vi "ACQUIS_BASE2_2015.vi"(1 "sample mode":i32(ring)=10178 items=["Finite Samples"=10178, "Continuous Samples"=10123, "Hardware Timed Single Point"=12522], 2 "Campioni al secondo":sgl=50000.0, 3 "Fondo Scala":enum16{"10", "5", "0.5", "0.05"}(ring), 4 "physical channels":tag="Dev1/ai0:1", 5 "input terminal configuration":i32(ring)=10083 items=["default"=-1, "RSE"=10083, "NRSE"=10078, "Differential"=10106, "Pseudodifferential"=12529], 6 "Durata (secondi)":dbl=0.05 format="%#.5f") -> ()   [LabVIEW 2014]
doc: "AnalogInput versione 7\nVersione base (2 canale) per schede 6024E\n(per le 6221 occorre cambiare il vettore Fondo scala)\nFM & ADL 2007\nsalva anche i dati (due colonne con solo Y1 e Y2 dopo una riga di intestazione\ngenn 2013"
uses:
  <vilib>/DAQmx/read.llb/DAQmx Read (Analog 2D DBL NChan NSamp).vi
  <vilib>/DAQmx/create/channels.llb/DAQmx Create Channel (AI-Voltage-Basic).vi
  <vilib>/DAQmx/configure/timing.llb/DAQmx Timing (Sample Clock).vi
  <vilib>/DAQmx/miscellaneous.llb/DAQmx Fill In Error Info.vi
panel:
  out "Grafico Dati":dbl[][](graph)
  in  "SALVA I DATI SU FILE":bool=TRUE caption="ON\nOFF"
  # "NO\nSI"
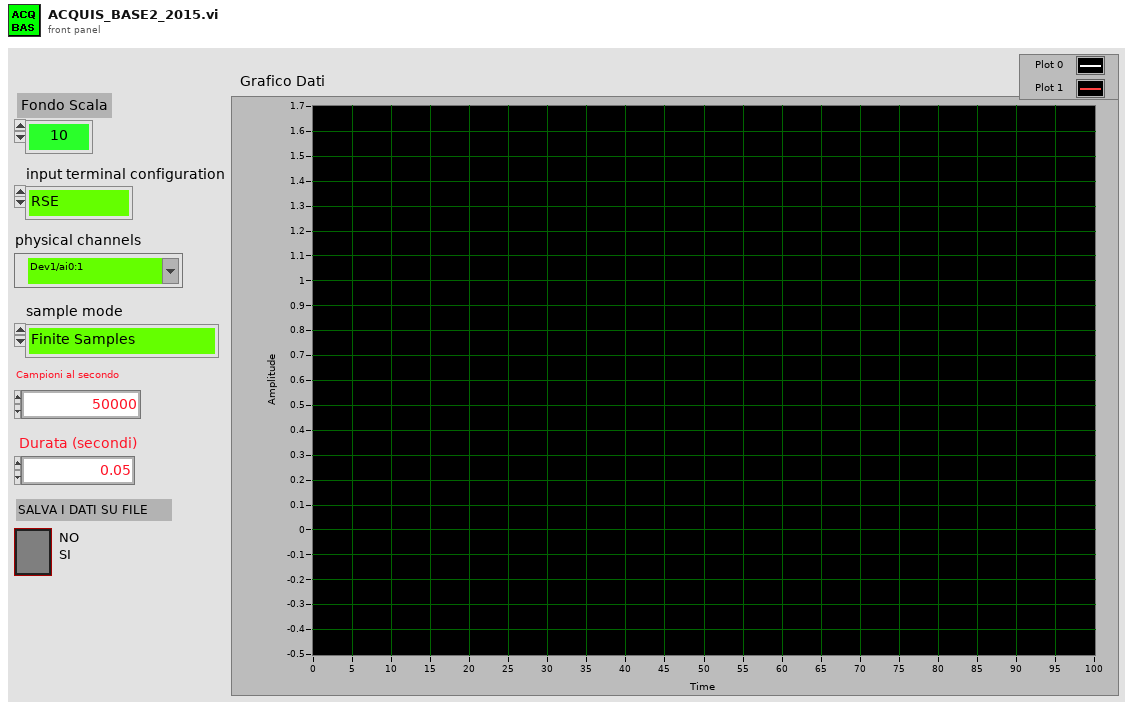
[diagram p1: front panel]
types:
  T1 = enum32{"existing file", "new file", "new or existing file", "existing dir", "new dir", "new or existing dir", "existing file (use LLBs)", "new file (use LLBs)", "new or existing file (use LLBs)", "new or existing file or directory (use LLBs)"}
  T2 = enum16{"open", "replace", "create", "open or create", "replace or create", "replace or create with confirmation"}
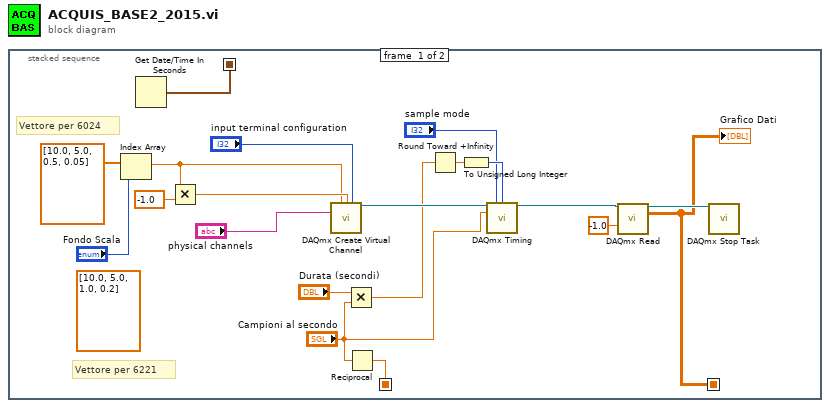
[diagram p0: block diagram]
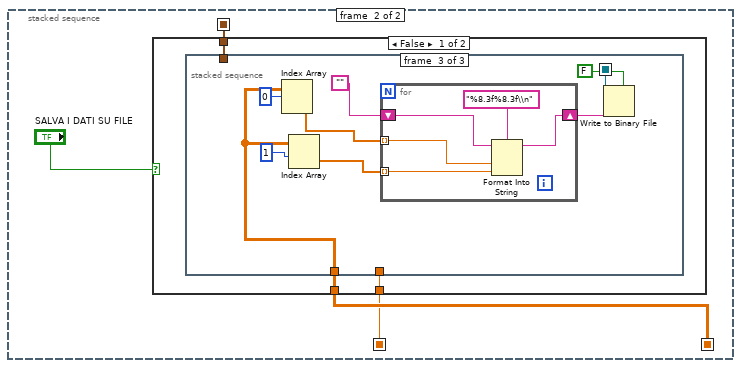
[diagram p2: hidden frame]
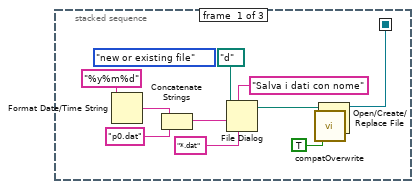
[diagram p3: hidden frame]
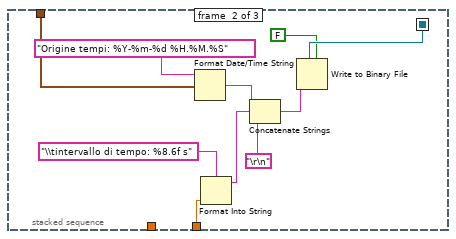
[diagram p4: hidden frame]
diagram:
  n1 = stacked-sequence {
    seq-local: [w4 _] -> [_ w23]
    seq-local: [w3 _] -> [_ w22]
    seq-local: [w1 _] -> [_ w21]
    frame #0 {
      (unwired) dbl[] [10.0, 5.0, 1.0, 0.2] ("Input Array")
      # "Vettore per 6024"
      # "Vettore per 6221"
      n2 = Index Array(array=dbl[] [10.0, 5.0, 0.5, 0.05] ("Input Array"), index="Fondo Scala") -> (element=w14:dbl)
      n3 = Get Date/Time In Seconds() -> (seconds since 1Jan1904=w3:timestamp)
      n4 = Multiply(x=w14, y=-1.0) -> (x*y=w15:dbl)
      n5 = call-poly <vilib>:"DAQmx Create Virtual Channel.vi"("maximum value"=w14, "minimum value"=w15, "input terminal configuration"="input terminal configuration", "physical channels"="physical channels") -> ("task out"=w13:refnum<k21>)  [unwired: 5 in, 6 out]
      n6 = Multiply(x="Durata (secondi)", y="Campioni al secondo") -> (x*y=w11:dbl)
      n7 = Reciprocal(x="Campioni al secondo") -> (1/x=w1:sgl)
      n8 = Round Toward +Infinity(x=w11) -> (ceil(x): smallest int >= x=w10:dbl)
      n9 = To Unsigned Long Integer(number=w10) -> (unsigned 32bit integer=w9:u32)
      n10 = call-poly <vilib>:"DAQmx Timing.vi"("task/channels in"=w13, "sample mode"="sample mode", "samples per channel"=w9, "rate"="Campioni al secondo") -> ("task out"=w7:refnum<k21>)  [unwired: 3 in, 8 out]
      n11 = call-poly <vilib>:"DAQmx Read.vi"("task/channels in"=w7, "timeout"=-1.0) -> ("task out"=w6:refnum<k21>, "data"=w4:dbl[][])  [unwired: 2 in, 10 out]
      "Grafico Dati" <- w4
      n12 = call <vilib>:"DAQmx Stop Task.vi"("task/channels in"=w6) -> ()  [unwired: 1 in, 14 out]
    }
    frame #1 {
      n13 = case shown="False" "SALVA I DATI SU FILE" {
        tunnel: w23 -> [w26 _]
        tunnel: w22 -> [w27 _]
        tunnel: w21 -> [w25 _]
        frame False {
          n14 = stacked-sequence {
            seq-local: [w29 _ _] -> [_ w47 w55]
            tunnel: w27 -> [_ w46 _]
            tunnel: w26 -> [_ _ w52]
            tunnel: w25 -> [_ w41 _]
            frame #0 {
              (unwired) T1."new or existing file" ("select mode (2)")
              n15 = Format Date/Time String(time format string (%c)="%y%m%d") -> (date/time string=w33:string)  [unwired: 2 out]
              n16 = Concatenate Strings(w33, "p0.dat") -> (w31:string)
              n17 = File Dialog(6:"*.dat", 7:"Salva i dati con nome", 9:w31, 11:path "d:/") -> (3:w38:path)  [unwired: 1 in, 5 out]
              n18 = call <vilib>:"compatOverwrite.vi"("overwrite (F)"=TRUE) -> ("overwrite?"=w28:T2)
              n19 = Open/Create/Replace File(file path (use dialog)=w38, operation (0:open)=w28) -> (refnum out=w29:refnum<file>)  [unwired: 1 in, 5 out]
            }
            frame #1 {
              n20 = Format Date/Time String(time format string (%c)="Origine tempi: %Y-%m-%d %H.%M.%S", seconds (now)=w46) -> (date/time string=w45:string)  [unwired: 1 out]
              n21 = Format Into String(format string="\\tintervallo di tempo: %8.6f s", w41) -> (resulting string=w40:string)  [unwired: 2 in, 1 out]
              n22 = Concatenate Strings(w45, w40, "\r\n") -> (w44:string)
              n23 = Write to Binary File(file (use dialog)=w47, data=w44, 5:FALSE ("prepend array or string size? (T)")) -> ()  [unwired: 1 in, 5 out]
            }
            frame #2 {
              n24 = Index Array(array=w52, index (row)=0 ("index")) -> (element=w53:dbl[])  [unwired: 1 in]
              n25 = Index Array(array=w52, index (row)=1 ("index")) -> (element=w50:dbl[])  [unwired: 1 in]
              n26 = for {
                shift-right: [w61] -> w57
                shift-left: "" -> [w60]
                tunnel: w53 -> [w59] mode=indexing
                tunnel: w50 -> [w58] mode=indexing
                n27 = Format Into String(format string="%8.3f%8.3f\\n" ("Format String"), initial string=w60, w59, w58) -> (resulting string=w61:string)  [unwired: 1 in, 1 out]
              }
              n28 = Write to Binary File(file (use dialog)=w55, data=w57, 5:FALSE ("prepend array or string size? (T)")) -> ()  [unwired: 1 in, 5 out]
            }
          }
        }
        frame True {
        }
      }
    }
  }
